vi "CMI ADS127L21 - Close.vi"(8 "error in (no error)":errorcluster, 10 "stop sampling? (False)":bool, 11 "session in":T1 {"channels"."Channel" min=1 max=8 step=1}) -> (0 "error out":errorcluster)   [LabVIEW 2020]
doc: "Close digitizer."
uses:
  CMI ADS127L21 - Session.ctl
  CMI ADS127L21 - Record Channel.ctl
  CMI ADS127L21 - Input Range.ctl
  CMI ADS127L21 - Input Mode.ctl
  CMI ADS127L21 - Input Impedance.ctl
  CMI ADS127L21 - EXTOUT Mode.ctl
  CMI ADS127L21 - EXTOUT Polarity.ctl
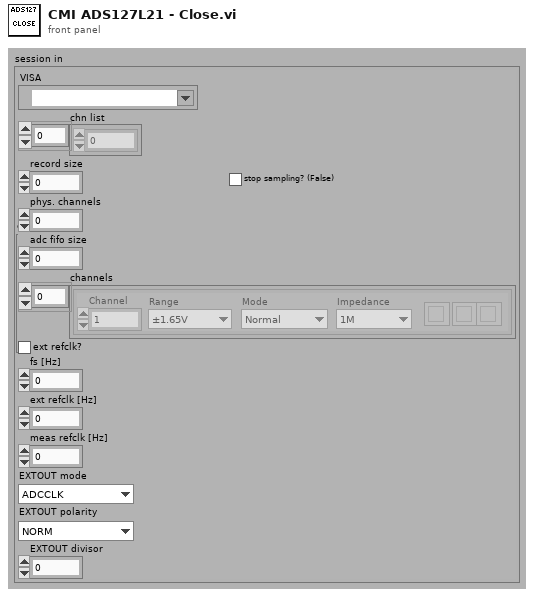
[diagram p1: front panel]
types:
  T1 = typedef "CMI ADS127L21 - Session.ctl" = cluster{"VISA":refnum<visa-resource-name>, "chn list":i32[], "record size":i32, "phys. channels":i32, "adc fifo size":i32, "channels":T2[], "ext refclk?":bool, "fs [Hz]":dbl, "ext refclk [Hz]":dbl, "meas refclk [Hz]":dbl, "EXTOUT mode":T6, "EXTOUT polarity":T7, "EXTOUT divisor":i32}
  T2 = typedef "CMI ADS127L21 - Record Channel.ctl" = cluster{"Range":T3, "Channel":i32, "Mode":T4, "Impedance":T5, "btn clr":bool, "btn up":bool, "btn down":bool}
  T3 = typedef "CMI ADS127L21 - Input Range.ctl" = enum16{"±1.65V", "±2V"}
  T4 = typedef "CMI ADS127L21 - Input Mode.ctl" = enum16{"Normal", "Inverted", "GND"}
  T5 = typedef "CMI ADS127L21 - Input Impedance.ctl" = enum16{"1M", "1k5"}
  T6 = typedef "CMI ADS127L21 - EXTOUT Mode.ctl" = enum16{"ADCCLK", "REFCLK", "SMPLCLK", "FIRST"}
  T7 = typedef "CMI ADS127L21 - EXTOUT Polarity.ctl" = enum16{"NORM", "INV"}
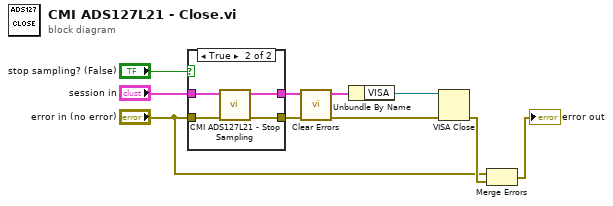
[diagram p0: block diagram]
diagram:
  n1 = case shown="True" "stop sampling? (False)" {
    tunnel: "error in (no error)" -> [w10 w15]
    tunnel: [w10 w14] -> w4
    tunnel: [w11 w13] -> w3
    tunnel: "session in" -> [w11 w12]
    frame False {
    }
    frame True {
      n2 = call "CMI ADS127L21 - Stop Sampling.vi"("error in (no error)"=w15, "session in"=w12) -> ("error out"=w14:errorcluster, "session out"=w13:T1)  [unwired: 8 in]
    }
  }
  n3 = call <vilib>:"Clear Errors.vi"("error in (no error)"=w4) -> ("error out"=w8:errorcluster)  [unwired: 5 in, 1 out]
  n4 = Unbundle By Name(w3) -> ("VISA"=w9:refnum<visa-resource-name>)
  n5 = VISA Close(VISA resource name=w9, error in (no error)=w8) -> (error out=w7:errorcluster)
  n6 = Merge Errors("error in (no error)", w7) -> (→"error out":errorcluster)
